vi "Socket Write.vi"(8 "error in (no error)":errorcluster, 9 "timeout ms (5000)":i32=5000, 10 "Bytes to write":u8[](array[numeric]), 11 "WebSocket in":refnum<class "WebSocket.lvclass">) -> (0 "error out":errorcluster, 2 "bytes written":i32, 3 "WebSocket out":refnum<class "WebSocket.lvclass">)   [LabVIEW 2013, in "WebSockets.lvlib" / "WebSocket.lvclass"]
uses:
  WebSocket.lvclass
  WebSocket.lvclass/WebSocket.ctl
  Sockets/Socket/Socket.lvclass
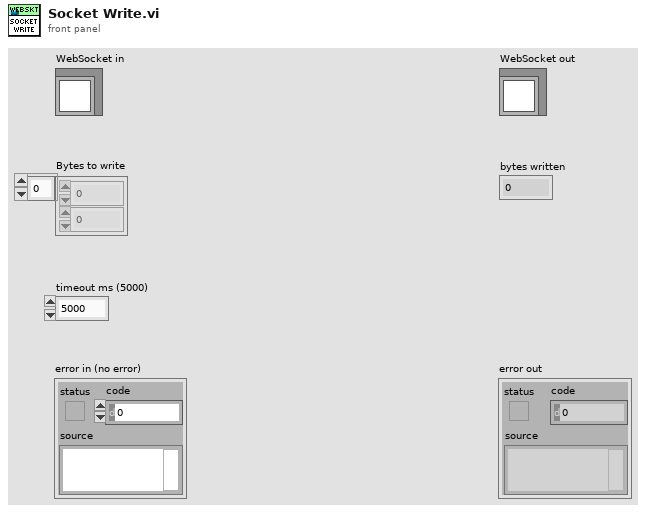
[diagram p1: front panel]
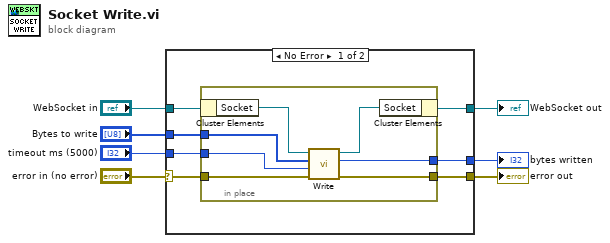
[diagram p0: block diagram]
diagram:
  n1 = case shown="No Error" "error in (no error)" {
    selector: "error in (no error)" -> [w11 w22]
    tunnel: [w8 w23] -> w5
    tunnel: "WebSocket in" -> [w14 w23]
    tunnel: "Bytes to write" -> [w13 _]
    tunnel: "timeout ms (5000)" -> [w12 _]
    tunnel: [w10 w22] -> w2
    tunnel: [w9 _] -> w1
    frame No Error {
      n2 = in-place {
        in-place-border: w13 -> [w20]
        in-place-border: w12 -> [w19]
        in-place-border: w11 -> [w18]
        in-place-border: [w17] -> w10
        in-place-border: [w16] -> w9
        n3 = in-place-cluster #1(w14) -> ("Socket"=w21:refnum<class "Socket.lvclass">)
        n4 = call-dynamic "Write.vi"("error in (no error)"=w18, "timeout ms (25000)"=w19, "Bytes to write"=w20, "Socket in"=w21) -> ("error out"=w17:errorcluster, "bytes written"=w16:i32, "Socket out"=w15:refnum<class "Socket.lvclass">)  [unwired: 5 in]
        n5 = in-place-cluster #1("Socket"=w15) -> (w8:refnum<class "WebSocket.lvclass">)
      }
    }
    frame Error {
    }
  }
  "error out" <- w2
  "WebSocket out" <- w5
  "bytes written" <- w1
